vi "GET USERS ITEMS.vi"(5 "DAYS BETWEEN REMINDERS":string, 7 "DAYS BEFORE DUE DATE":string, 10 "BYU ID # IN":string, 11 "connection reference in":T3) -> (1 "DATA OUT":T2, 3 "connection reference out":T3)   [LabVIEW 2019]
uses:
  <vilib>/addons/database/Connection.llb/Conn ObjectReference.ctl
  Controls/Table Data Types/Inventory Data Type.ctl
  <vilib>/addons/database/Auxilliary.llb/DB Tools Cursor Type.ctl
  <vilib>/addons/database/Connection.llb/Conn Execute.vi
  <vilib>/addons/database/Recordset.llb/Rec Fetch Recordset Data (R).vi
  <vilib>/addons/database/Recordset.llb/Rec Destroy - Connection.vi
  <vilib>/addons/database/_DB Variant To Data/Database Variant To Data.xnode
  <vilib>/addons/database/NI_Database_API.lvlib
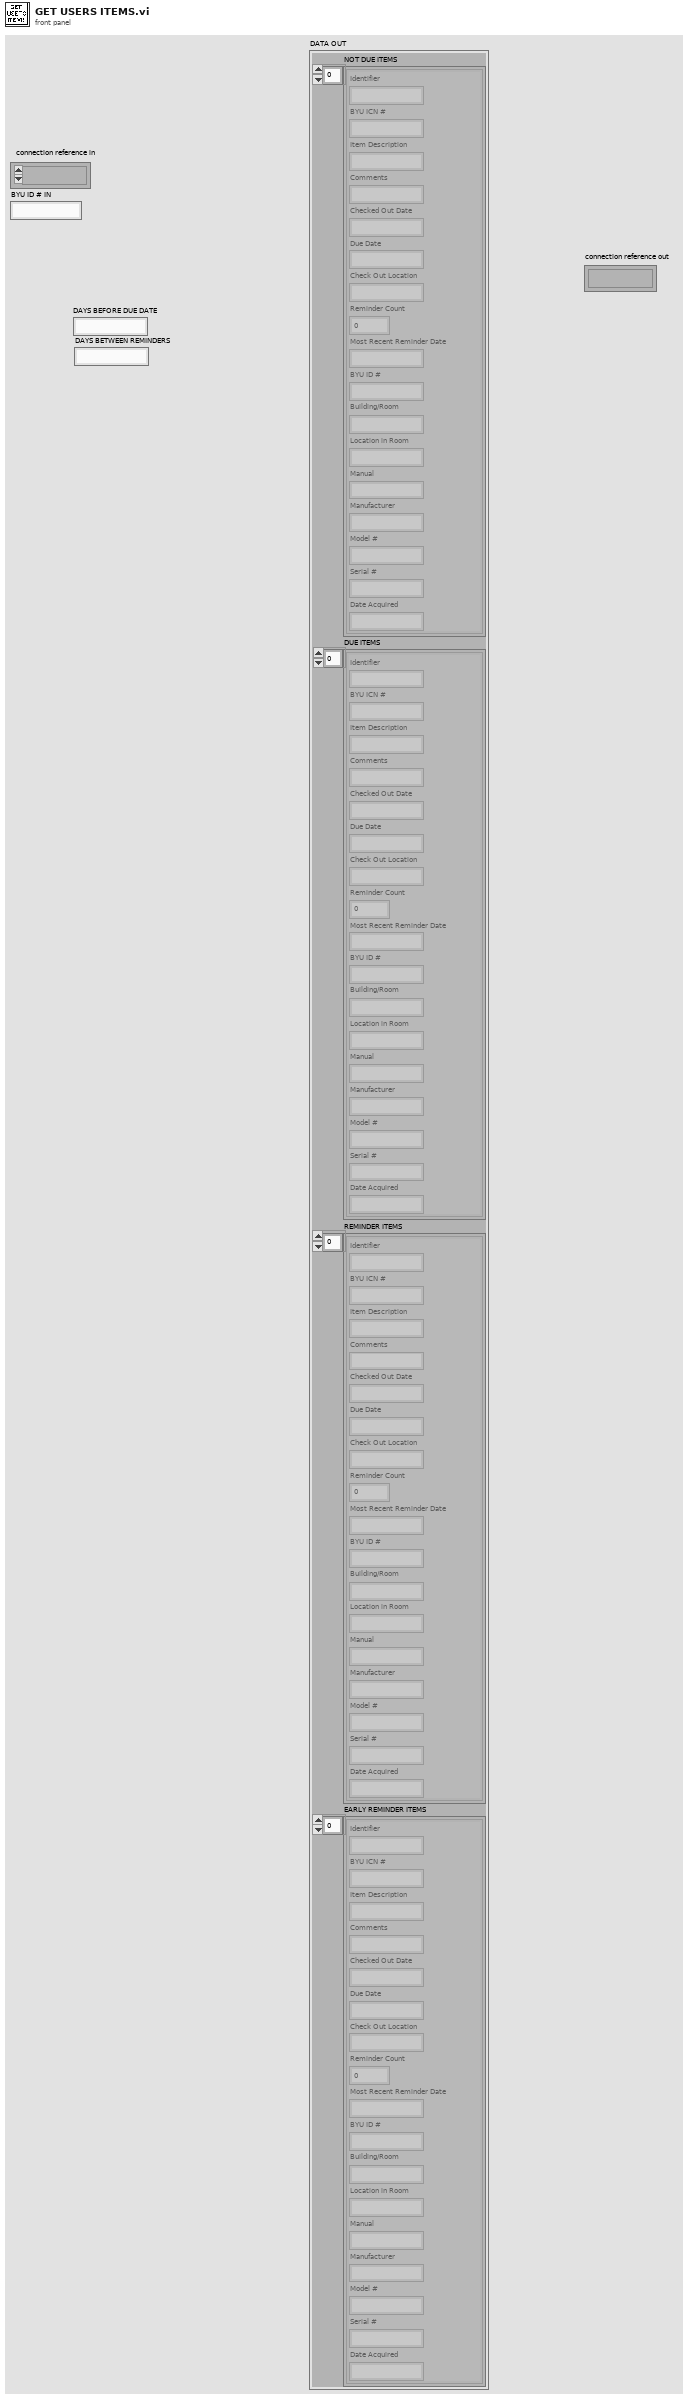
[diagram p1: front panel]
types:
  T1 = typedef "Inventory Data Type.ctl" = cluster{"Identifier":string, "BYU ICN #":string, "Item Description":string, "Comments":string, "Checked Out Date":string, "Due Date":string, "Check Out Location":string, "Reminder Count":i32, "Most Recent Reminder Date":string, "BYU ID #":string, "Building/Room":string, "Location in Room":string, "Manual":string, "Manufacturer":string, "Model #":string, "Serial #":string, "Date Acquired":string}
  T2 = cluster{"NOT DUE ITEMS":T1[], "DUE ITEMS":T1[], "REMINDER ITEMS":T1[], "EARLY REMINDER ITEMS":T1[]}
  T3 = typedef "NI_Database_API.lvlib/Conn ObjectReference.ctl" = refnum<k1>
  T4 = typedef "NI_Database_API.lvlib/DB Tools Cursor Type.ctl" = enum16{"forward-only", "keyset", "dynamic", "static"}
  T5 = typedef "NI_Database_API.lvlib/Rec ObjectReference.ctl" = refnum<k1>
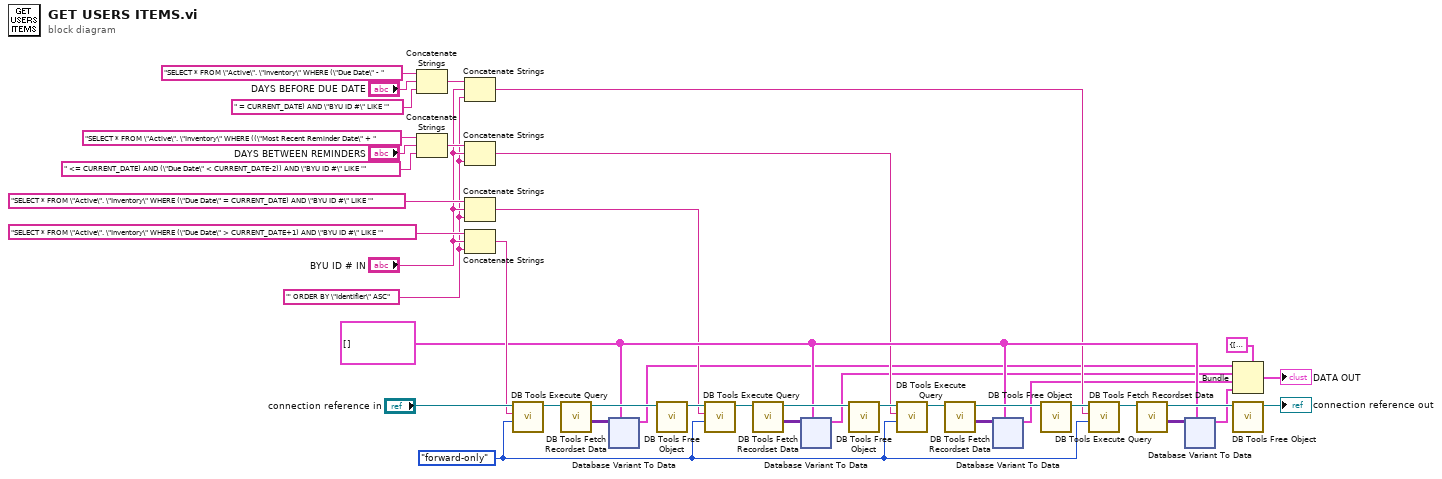
[diagram p0: block diagram]
diagram:
  w10 = DB_Tools_Cursor_Type."forward-only" ("cursor type")
  w30 = "' ORDER BY \"Identifier\" ASC"
  w12 = T1[] [] ("Array")
  n1 = Concatenate Strings("SELECT * FROM \"Active\". \"Inventory\" WHERE (\"Due Date\" - ", "DAYS BEFORE DUE DATE", " = CURRENT_DATE) AND \"BYU ID #\" LIKE '") -> (w35:string)
  n2 = Concatenate Strings("SELECT * FROM \"Active\". \"Inventory\" WHERE ((\"Most Recent Reminder Date\" + ", "DAYS BETWEEN REMINDERS", " <= CURRENT_DATE) AND (\"Due Date\" < CURRENT_DATE-2)) AND \"BYU ID #\" LIKE '") -> (w34:string)
  n3 = Concatenate Strings(w35, "BYU ID # IN", w30) -> (w8:string)
  n4 = Concatenate Strings(w34, "BYU ID # IN", w30) -> (w9:string)
  n5 = Concatenate Strings("SELECT * FROM \"Active\". \"Inventory\" WHERE (\"Due Date\" = CURRENT_DATE) AND \"BYU ID #\" LIKE '", "BYU ID # IN", w30) -> (w11:string)
  n6 = Concatenate Strings("SELECT * FROM \"Active\". \"Inventory\" WHERE (\"Due Date\" > CURRENT_DATE+1) AND \"BYU ID #\" LIKE '", "BYU ID # IN", w30) -> (w28:string)
  n7 = call-poly <vilib>:"DB Tools Execute Query.vi"("cursor type"=w10, "SQL query"=w28, "connection reference"="connection reference in") -> ("recordset reference"=w27:T5)  [unwired: 5 in, 1 out]
  n8 = call-poly <vilib>:"DB Tools Fetch Recordset Data.vi"("recordset reference"=w27) -> ("recordset data"=w25:variant[][], "recordset reference out"=w26:T5)  [unwired: 4 in, 1 out]
  n9 = xnode "Database Variant To Data"("database variant"=w25, "type"=w12) -> ("data"=w1:T1[])  [unwired: 1 in, 1 out]
  n10 = call-poly <vilib>:"DB Tools Free Object.vi"("recordset reference"=w26) -> ("connection reference"=w21:T3)  [unwired: 9 in, 1 out]
  n11 = call-poly <vilib>:"DB Tools Execute Query.vi"("cursor type"=w10, "SQL query"=w11, "connection reference"=w21) -> ("recordset reference"=w22:T5)  [unwired: 5 in, 1 out]
  n12 = call-poly <vilib>:"DB Tools Fetch Recordset Data.vi"("recordset reference"=w22) -> ("recordset data"=w24:variant[][], "recordset reference out"=w23:T5)  [unwired: 4 in, 1 out]
  n13 = xnode "Database Variant To Data"("database variant"=w24, "type"=w12) -> ("data"=w2:T1[])  [unwired: 1 in, 1 out]
  n14 = call-poly <vilib>:"DB Tools Free Object.vi"("recordset reference"=w23) -> ("connection reference"=w17:T3)  [unwired: 9 in, 1 out]
  n15 = call-poly <vilib>:"DB Tools Execute Query.vi"("cursor type"=w10, "SQL query"=w9, "connection reference"=w17) -> ("recordset reference"=w20:T5)  [unwired: 5 in, 1 out]
  n16 = call-poly <vilib>:"DB Tools Fetch Recordset Data.vi"("recordset reference"=w20) -> ("recordset data"=w18:variant[][], "recordset reference out"=w19:T5)  [unwired: 4 in, 1 out]
  n17 = xnode "Database Variant To Data"("database variant"=w18, "type"=w12) -> ("data"=w3:T1[])  [unwired: 1 in, 1 out]
  n18 = call-poly <vilib>:"DB Tools Free Object.vi"("recordset reference"=w19) -> ("connection reference"=w13:T3)  [unwired: 9 in, 1 out]
  n19 = call-poly <vilib>:"DB Tools Execute Query.vi"("cursor type"=w10, "SQL query"=w8, "connection reference"=w13) -> ("recordset reference"=w14:T5)  [unwired: 5 in, 1 out]
  n20 = call-poly <vilib>:"DB Tools Fetch Recordset Data.vi"("recordset reference"=w14) -> ("recordset data"=w16:variant[][], "recordset reference out"=w15:T5)  [unwired: 4 in, 1 out]
  n21 = xnode "Database Variant To Data"("database variant"=w16, "type"=w12) -> ("data"=w4:T1[])  [unwired: 1 in, 1 out]
  n22 = Bundle(cluster=T2 {"NOT DUE ITEMS"=[], "DUE ITEMS"=[], "REMINDER ITEMS"=[], "EARLY REMINDER ITEMS"=[]} ("EMAIL ITEMS"), "NOT DUE ITEMS"=w1, "DUE ITEMS"=w2, "REMINDER ITEMS"=w3, "EARLY REMINDER ITEMS"=w4) -> (→"DATA OUT":T2)
  n23 = call-poly <vilib>:"DB Tools Free Object.vi"("recordset reference"=w15) -> ("connection reference"=→"connection reference out":T3)  [unwired: 9 in, 1 out]
